vi "sub_findMissingNumbersAndIndexes.vi"(8 "error in (no error)":errorcluster, 11 "row (in)":string[](array[string])) -> (0 "error out":errorcluster, 1 "row solved":bool, 3 "missing numbers":string[](array[string]))   [LabVIEW 2018]
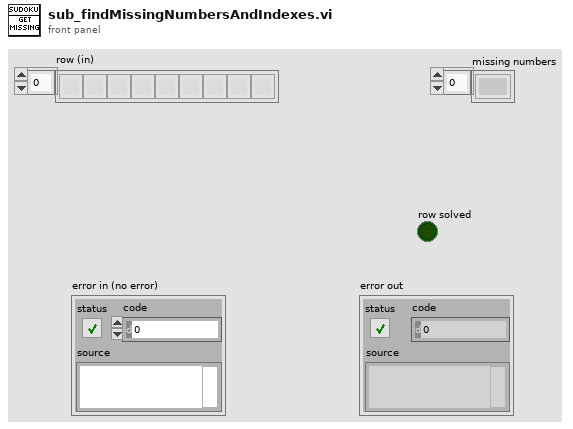
[diagram p1: front panel]
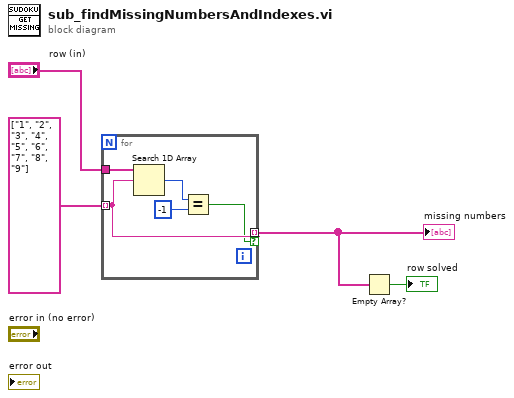
[diagram p0: block diagram]
diagram:
  n1 = for {
    tunnel: string[] ["1", "2", "3", "4", "5", "6", "7", "8", "9"] -> [w6] mode=indexing
    tunnel: "row (in)" -> [w9]
    tunnel: [w6] -> w2 mode=indexing if=w5
    n2 = Search 1D Array(1D array=w9, element=w6) -> (index of element=w8:i32)  [unwired: 1 in]
    n3 = Equal?(x=w8, y=-1) -> (x = y?=w5:bool)
  }
  "missing numbers" <- w2
  n4 = Empty Array?(array=w2) -> (empty?=→"row solved":bool)
